vi "Controller_Geared_Template.vi"() -> ()   [LabVIEW 2017]
uses:
  <vilib>/addons/control/pid/NI_PID_pid.lvlib
  <vilib>/platform/TimedLoop/XDataNode/XDataNode.xnode
  <vilib>/Platform/TimedLoop/XDataNode/nitl_modes.ctl
  <vilib>/Platform/TimedLoop/XDataNode/XDNodeRunTimeDep.lvlib
  <vilib>/Platform/TimedLoop/XDataNode/wakeup.ctl
  <vilib>/Platform/TimedLoop/XDataNode/timing_clust.ctl
  <vilib>/addons/control/pid/_prctrl compat.llb/PID (Compatibility).vi
  <vilib>/addons/control/pid/NI_PID__prctrl compat.lvlib
panel:
  out "Actuation Maximum":dbl(slide) scale=0.0..100.0
  in  "Controller\nReset":bool
  in  "Setpoint":dbl
  out "Actuation":dbl
  out "Fault":bool
  in  "Controller":string(combo)
  in  "stop":bool
  # "IHX Control"
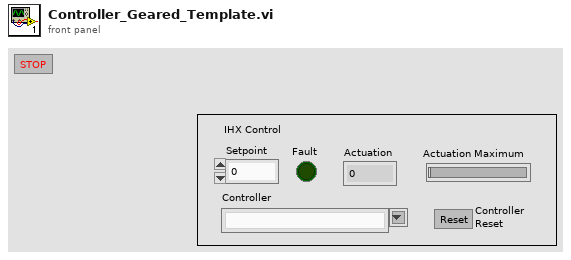
[diagram p1: front panel]
types:
  T1 = typedef "XDNodeRunTimeDep.lvlib/timing_clust.ctl" = cluster{"Expected End [f-1]":u64, "Actual End [f-1]":u64, "Finished Late? [f-1]":bool, "Expected End [i-1]":u64, "Actual End [i-1]":u64, "Finished Late? [i-1]":bool, "Expected Start [i]":u64, "Actual Start [i]":u64, "Expected Start [f]":u64, "Actual Start [f]":u64, "Source Name":string, "Structure Name":string, "Period":i64, "Deadline":i64, "Offset":i64, "Start":i64, "Priority":i32, "Timeout":i32, "Mode":T2, "Wakeup Reason":T3, "Error":errorcluster, "Source Type":string, "Secondary Source Type":string, "Global End Time":u64, "Global Start Time":u64, "Frame Duration":u64, "Iteration Duration":u64, "Assigned CPU":i32, "I/O Scan Engine Mode":u32}
  T2 = typedef "XDNodeRunTimeDep.lvlib/nitl_modes.ctl" = enum32{"No Change", "Process missed periods, maintain original phase", "Discard missed periods, maintain original phase", "Process missed periods, ignore original phase", "Discard missed periods, ignore original phase"}
  T3 = typedef "XDNodeRunTimeDep.lvlib/wakeup.ctl" = enum32{"Normal", "Aborted", "Asynchronous wakeup", "Timing source error", "Timed loop error", "Timeout"}
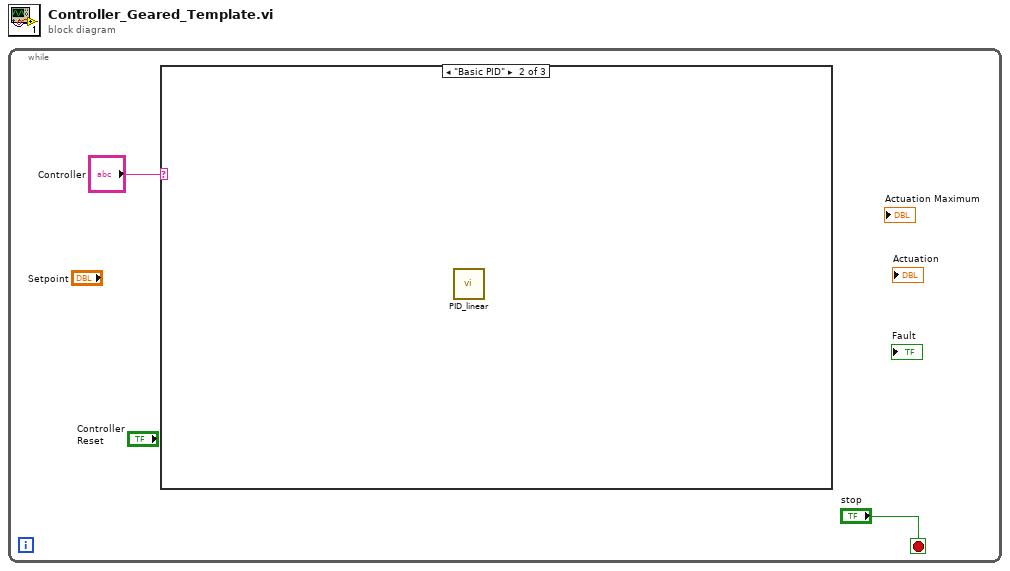
[diagram p0: block diagram]
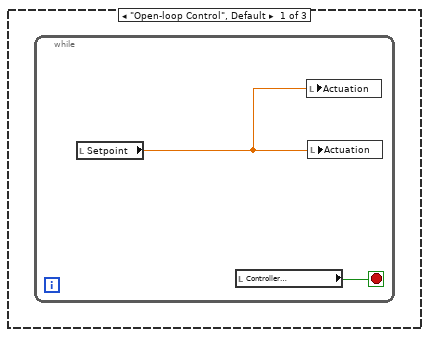
[diagram p2: hidden frame]
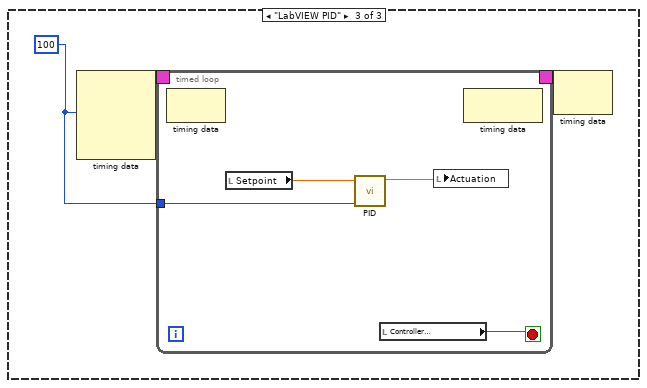
[diagram p3: hidden frame]
diagram:
  n1 = while {
    stop <- "stop" stop-if-true
    n2 = case shown="\"Basic PID\"" "Controller" {
      frame "Open-loop Control", Default {
        n3 = while {
          stop <- w3 stop-if-true
          n4 = local read "Setpoint"() -> (w4:dbl)
          n5 = local read "Controller\nReset"() -> (w3:bool)
          n6 = local write "Actuation"(w4) -> ()
          n7 = local write "Actuation"(w4) -> ()
        }
      }
      frame "Basic PID" {
        n8 = call "PID_linear.vi"() -> ()  [unwired: 12 in]
      }
      frame "LabVIEW PID" {
        w5 = 100
        n9 = node-c288(w5) -> (w7:T1)  [unwired: 3 in]
        n10 = timed-loop {
          timing: w7 -> [_]
          timing-out: [_] -> w6
          tunnel: w5 -> [w8]
          stop <- w11 stop-if-true
          n11 = node-c288() -> ()  [unwired: 1 in, 1 out]
          n12 = local read "Setpoint"() -> (w10:dbl)
          n13 = call-poly <vilib>:"PID.vi"("manual control"=w8, "setpoint"=w10) -> ("output"=w9:dbl)  [unwired: 9 in]
          n14 = local read "Controller\nReset"() -> (w11:bool)
          n15 = local write "Actuation"(w9) -> ()
          n16 = node-c288() -> ()  [unwired: 1 in, 1 out]
        }
        n17 = node-c288(w6) -> ()  [unwired: 1 out]
      }
    }
  }
